vi "Garbage.vi"() -> ()   [LabVIEW 2011]
panel:
  in  "Abort":bool
  in  "Begin":bool
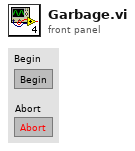
[diagram p1: front panel]
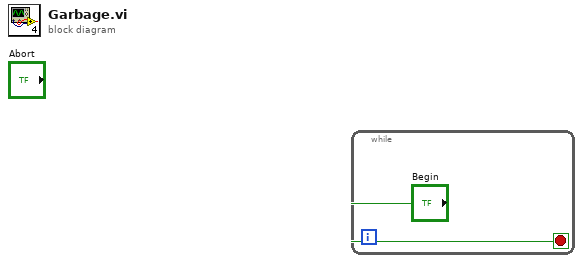
[diagram p0: block diagram]
diagram:
  n1 = while {
    stop <- "Begin" stop-if-true
  }
